vi "tra25cc_stop.vi"(8 "error in (no error)":errorcluster, 11 "conn_xyz_in":T2) -> (0 "error out":errorcluster, 3 "conn_xyz_out":T1)   [LabVIEW 2014]
uses:
  \\CL3-USR4\usr4/F103625/Scanner_v3_current/src/Stage_xyz/Dll/Newport.CONEXCC.CommandInterface.dll
  Dll/Newport.CONEXCC.CommandInterface.dll
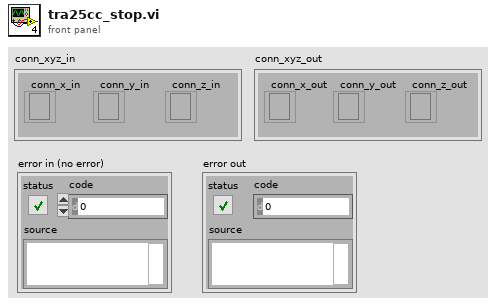
[diagram p1: front panel]
types:
  T1 = cluster{"conn_x_out":refnum<k24>, "conn_y_out":refnum<k24>, "conn_z_out":refnum<k24>}
  T2 = cluster{"conn_x_in":refnum<k24>, "conn_y_in":refnum<k24>, "conn_z_in":refnum<k24>}
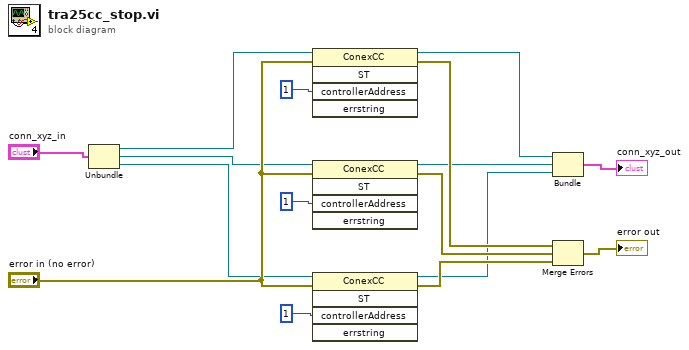
[diagram p0: block diagram]
diagram:
  n1 = Unbundle("conn_xyz_in") -> ("conn_x_in"=w10:refnum<k24>, "conn_y_in"=w9:refnum<k24>, "conn_z_in"=w8:refnum<k24>)
  n2 = invoke class="ConexCC" method="ST"(reference=w10, error in="error in (no error)", "controllerAddress"=1) -> (reference out=w6:refnum<k24>, error out=w12:errorcluster)  [unwired: 2 in, 3 out]
  n3 = invoke class="ConexCC" method="ST"(reference=w9, error in="error in (no error)", "controllerAddress"=1) -> (reference out=w5:refnum<k24>, error out=w13:errorcluster)  [unwired: 2 in, 3 out]
  n4 = invoke class="ConexCC" method="ST"(reference=w8, error in="error in (no error)", "controllerAddress"=1) -> (reference out=w4:refnum<k24>, error out=w14:errorcluster)  [unwired: 2 in, 3 out]
  n5 = Bundle("conn_x_in"=w6, "conn_y_in"=w5, "conn_z_in"=w4) -> (→"conn_xyz_out":T2)  [unwired: 1 in]
  n6 = Merge Errors(w12, w13, w14) -> (→"error out":errorcluster)
